vi "Open Sequence File.vi"(0 "Session Handle in":T3, 1 "Load Options":T2={"Use Search Dirs? (T)"=TRUE, "Conflict as Error? (T)"=TRUE, "Check Station Model? (F)"=FALSE, "Preload Modules? (T)"=TRUE, "Skip Load Callback? (F)"=FALSE, "Reload if Loaded? (F)"=FALSE}, 5 "File Path":string, 9 "Current Seq File (None)":T1, 11 "error in (no error)":errorcluster) -> (4 "Session Handle out":T3, 6 "SequenceFile":T1, 15 "error out":errorcluster)   [LabVIEW 2020, in "HTS.lvlib" / "Engine.lvclass"]
uses:
  Engine.lvclass
  Typedefs/Session Handle.ctl
  SequenceFile/Typedefs/Session Handle.ctl
  SequenceFile/SequenceFile.lvclass
  Data Types/File Load Options.ctl
  Engine.lvclass/Engine.ctl
  HTS.lvlib
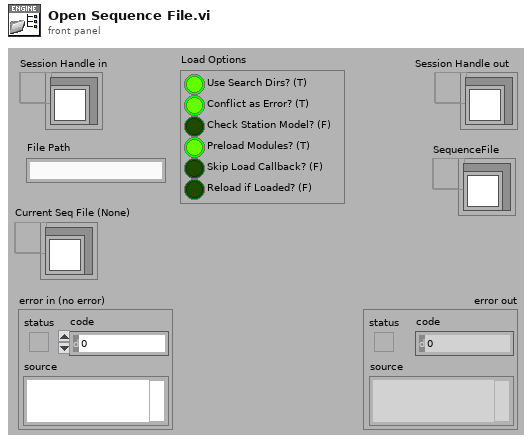
[diagram p1: front panel]
types:
  T1 = typedef "HTS.lvlib/SequenceFile.lvclass/Session Handle.ctl" = refnum<data-value>
  T2 = typedef "HTS.lvlib/File Load Options.ctl" = cluster{"Use Search Dirs? (T)":bool, "Conflict as Error? (T)":bool, "Check Station Model? (F)":bool, "Preload Modules? (T)":bool, "Skip Load Callback? (F)":bool, "Reload if Loaded? (F)":bool}
  T3 = typedef "HTS.lvlib/Engine.lvclass/Session Handle.ctl" = refnum<data-value>
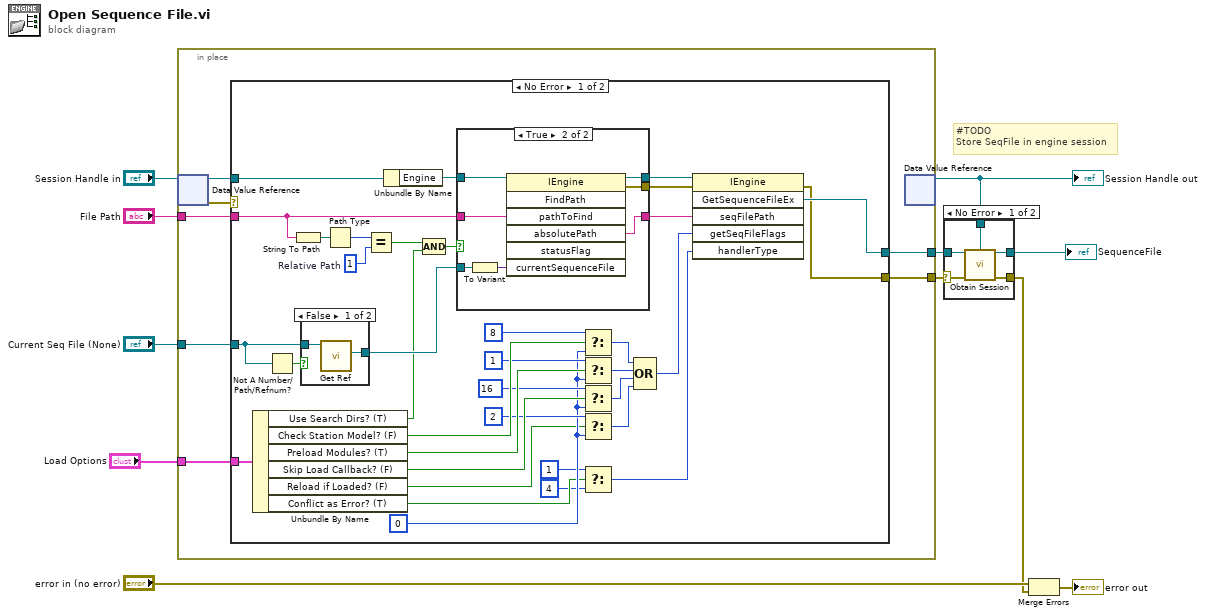
[diagram p0: block diagram]
diagram:
  # "#TODO\nStore SeqFile in engine session"
  n1 = in-place {
    in-place-border: "File Path" -> [w16]
    in-place-border: "Current Seq File (None)" -> [w15]
    in-place-border: "Load Options" -> [w14]
    in-place-border: [w13] -> w2
    in-place-border: [w12] -> w1
    n2 = in-place-dvr #1("Session Handle in") -> (w17:refnum<class "Engine.lvclass">, w18:errorcluster)
    n3 = case shown="No Error" w18 {
      selector: w18 -> [_ w66]
      tunnel: w17 -> [w54 _]
      tunnel: w16 -> [w47 _]
      tunnel: w15 -> [w44 _]
      tunnel: w14 -> [w41 _]
      tunnel: [w19 w66] -> w12
      tunnel: [w20 _] -> w13
      frame No Error {
        w32 = 0 ("getSeqFileFlags")
        w50 = i16 1  # Relative Path
        n4 = Unbundle By Name(w41) -> ("Use Search Dirs? (T)"=w40:bool, "Check Station Model? (F)"=w39:bool, "Preload Modules? (T)"=w37:bool, "Skip Load Callback? (F)"=w34:bool, "Reload if Loaded? (F)"=w31:bool, "Conflict as Error? (T)"=w29:bool)
        n5 = Not A Number/Path/Refnum?(number/path/refnum=w44) -> (NaN/Path/Refnum?=w45:bool)
        n6 = String To Path(string=w47) -> (path=w52:path)
        n7 = case shown="False" w45 {
          tunnel: w44 -> [w56 _]
          tunnel: [w55 _] -> w43
          frame False {
            n8 = call "Get Ref.vi"("Session Handle in"=w56) -> ("Ref"=w55:refnum<k7>)  [unwired: 8 in, 2 out]
          }
          frame True {
          }
        }
        n9 = Path Type(1:w52) -> (0:w51:i16)
        n10 = Equal?(x=w51, y=w50) -> (x = y?=w48:bool)
        n11 = Unbundle By Name(w54) -> ("Engine"=w53:refnum<k7>)
        n12 = Compound Arithmetic op=AND(w48, w40) -> (w49:bool)
        n13 = case shown="True" w49 {
          tunnel: w53 -> [w57 w65]
          tunnel: w47 -> [w58 w64]
          tunnel: [w58 w63] -> w42
          tunnel: [w57 w62] -> w46
          tunnel: w43 -> [_ w61]
          tunnel: [_ w59] -> w21
          frame False {
          }
          frame True {
            n14 = To Variant(anything=w61) -> (Variant=w60:variant)
            n15 = invoke class="IEngine" method="FindPath"(reference=w65, "pathToFind"=w64, "currentSequenceFile"=w60) -> (reference out=w62:refnum<k7>, error out=w59:errorcluster, "absolutePath"=w63:string)  [unwired: 4 in, 4 out]
          }
        }
        n16 = Select(t=8 ("getSeqFileFlags"), s=w39, f=w32) -> (s? t:f=w25:i32)
        n17 = Select(t=1 ("getSeqFileFlags"), s=w37, f=w32) -> (s? t:f=w26:i32)
        n18 = Select(t=16 ("getSeqFileFlags"), s=w34, f=w32) -> (s? t:f=w24:i32)
        n19 = Select(t=2 ("getSeqFileFlags"), s=w31, f=w32) -> (s? t:f=w23:i32)
        n20 = Select(t=1 ("getSeqFileFlags"), s=w29, f=4 ("getSeqFileFlags")) -> (s? t:f=w27:i32)
        n21 = Compound Arithmetic op=OR(w25, w26, w24, w23) -> (w22:i32)
        n22 = invoke class="IEngine" method="GetSequenceFileEx"(reference=w46, error in=w21, "seqFilePath"=w42, "getSeqFileFlags"=w22, "handlerType"=w27) -> (error out=w19:errorcluster, "GetSequenceFileEx"=w20:refnum<k7>)  [unwired: 1 in, 4 out]
      }
      frame Error {
      }
    }
    n23 = in-place-dvr #1() -> (w3:T3)  [unwired: 1 in, 1 out]
  }
  "Session Handle out" <- w3
  n24 = case shown="No Error" w1 {
    selector: w1 -> [w67 w72]
    tunnel: [w71 _] -> w5
    tunnel: [w70 w72] -> w4
    tunnel: w3 -> [w69 _]
    tunnel: w2 -> [w68 _]
    frame No Error {
      n25 = call "Obtain Session.vi"("SequenceFile"=w68, "Engine"=w69, "error in (no error)"=w67) -> ("Session Handle"=w71:T1, "error out"=w70:errorcluster)  [unwired: 11 in]
    }
    frame Error {
    }
  }
  "SequenceFile" <- w5
  n26 = Merge Errors("error in (no error)", w4) -> (→"error out":errorcluster)
